vi "data_combinate.vi"(8 "error in (no error)":errorcluster caption="错误输入（无错误）", 10 "data_in":T1={"PW"="", "MN"="", "table输入"="心跳包", "数据发送次数"=0, "枚举"=enum."返回请求应答", "type"="", "因子编码&数据类型"=[]}, 11 "data":string[][](array[string])) -> (0 "error out":errorcluster caption="错误输出", 3 "message":string)   [LabVIEW 2016, in "潮位站数据传输.lvlib"]
uses:
  HJ212/HJ212.lvclass
  data_combination/data_combination.lvclass/data_combination.ctl
  data_combination/data_combination.lvclass
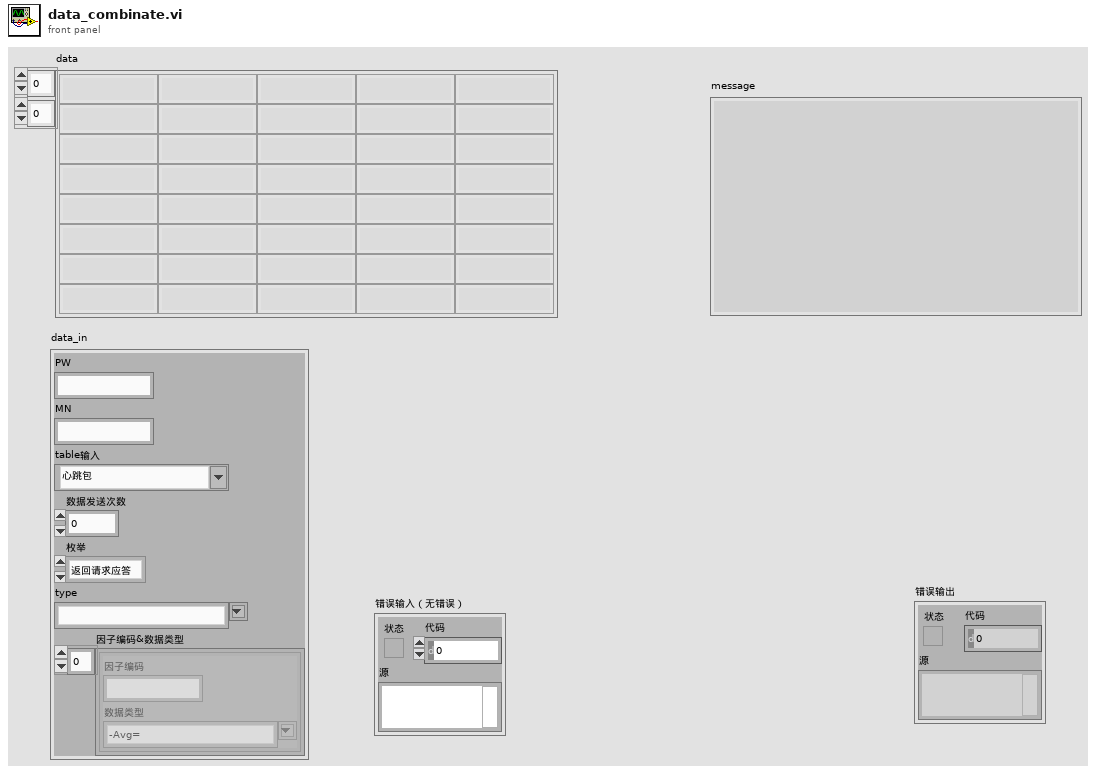
[diagram p1: front panel]
types:
  T1 = typedef "潮位站数据传输.lvlib/data_in.ctl" = cluster{"PW":string, "MN":string, "table输入":T2, "数据发送次数":i32, "枚举":enum16{"返回请求应答", "上传数据", "返回执行结果"}, "type":T3, "因子编码&数据类型":cluster{"因子编码":string, "数据类型":T4}[]}
  T2 = typedef "潮位站数据传输.lvlib/table.ctl" = string
  T3 = typedef "潮位站数据传输.lvlib/Type.ctl" = string
  T4 = typedef "潮位站数据传输.lvlib/data_type.ctl" = string
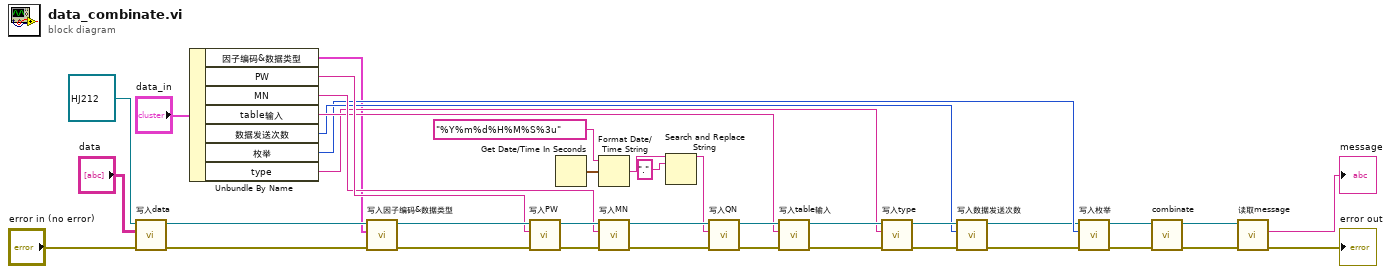
[diagram p0: block diagram]
diagram:
  n1 = call "写入data.vi"("error in (no error)"="error in (no error)", "data"="data", "data_combination输入"=refnum<class "HJ212.lvclass"> refnum ("HJ212.lvclass")) -> ("error out"=w28:errorcluster, "data_combination输出"=w31:refnum<class "HJ212.lvclass">)  [unwired: 7 in]
  n2 = Unbundle By Name("data_in") -> ("因子编码&数据类型"=w1:cluster{"因子编码":string, "数据类型":T4}[], "PW"=w11:string, "MN"=w10:string, "table输入"=w9:T2, "数据发送次数"=w8:i32, "枚举"=w6:enum16{"返回请求应答", "上传数据", "返回执行结果"}, "type"=w7:T3)
  n3 = call "写入因子编码&数据类型.vi"("error in (no error)"=w28, "因子编码&数据类型"=w1, "data_combination输入"=w31) -> ("error out"=w27:errorcluster, "data_combination输出"=w30:refnum<class "HJ212.lvclass">)  [unwired: 7 in]
  n4 = call "写入PW.vi"("error in (no error)"=w27, "PW"=w11, "data_combination输入"=w30) -> ("error out"=w26:errorcluster, "data_combination输出"=w36:refnum<class "HJ212.lvclass">)  [unwired: 7 in]
  n5 = Get Date/Time In Seconds() -> (seconds since 1Jan1904=w17:timestamp)
  n6 = Format Date/Time String(time format string (%c)="%Y%m%d%H%M%S%3u" ("时间格式字符串(%c)"), seconds (now)=w17) -> (date/time string=w16:string)  [unwired: 1 in]
  n7 = call "写入MN.vi"("error in (no error)"=w26, "MN"=w10, "data_combination输入"=w36) -> ("error out"=w25:errorcluster, "data_combination输出"=w35:refnum<class "HJ212.lvclass">)  [unwired: 7 in]
  n8 = Search and Replace String(input string=w16, search string="." ("搜索字符串")) -> (result string=w14:string)  [unwired: 6 in, 3 out]
  n9 = call "写入QN.vi"("error in (no error)"=w25, "QN"=w14, "data_combination输入"=w35) -> ("error out"=w24:errorcluster, "data_combination输出"=w34:refnum<class "HJ212.lvclass">)  [unwired: 7 in]
  n10 = call "写入table输入.vi"("error in (no error)"=w24, "table输入"=w9, "data_combination输入"=w34) -> ("error out"=w23:errorcluster, "data_combination输出"=w33:refnum<class "HJ212.lvclass">)  [unwired: 7 in]
  n11 = call "写入type.vi"("error in (no error)"=w23, "type"=w7, "data_combination输入"=w33) -> ("error out"=w22:errorcluster, "data_combination输出"=w32:refnum<class "HJ212.lvclass">)  [unwired: 7 in]
  n12 = call "写入数据发送次数.vi"("error in (no error)"=w22, "数据发送次数"=w8, "data_combination输入"=w32) -> ("error out"=w2:errorcluster, "data_combination输出"=w3:refnum<class "HJ212.lvclass">)  [unwired: 7 in]
  n13 = call "写入枚举.vi"("error in (no error)"=w2, "枚举"=w6, "data_combination输入"=w3) -> ("error out"=w21:errorcluster, "data_combination输出"=w29:refnum<class "HJ212.lvclass">)  [unwired: 7 in]
  n14 = call-dynamic "combinate.vi"("error in (no error)"=w21, "HJ212 输入"=w29) -> ("error out"=w20:errorcluster, "HJ212 输出"=w37:refnum<class "HJ212.lvclass">)  [unwired: 8 in]
  n15 = call "读取message.vi"("error in (no error)"=w20, "data_combination输入"=w37) -> ("error out"=→"error out":errorcluster, "message"=→"message":string)  [unwired: 7 in, 1 out]
